vi "toml_api_dump.vi"(7 "resolved path":path, 8 "error in (no error)":errorcluster, 10 "operation (open or create)":T1(ring)=enum."replace or create", 11 "vi in":refnum<vi>) -> (0 "error out":errorcluster, 2 "key exists":bool, 3 "vi out":refnum<vi>)   [LabVIEW 2017]
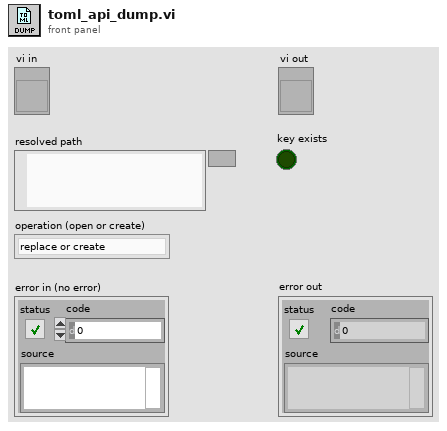
[diagram p1: front panel]
types:
  T1 = enum16{"open", "replace", "create", "open or create", "replace or create", "replace or create with confirmation"}
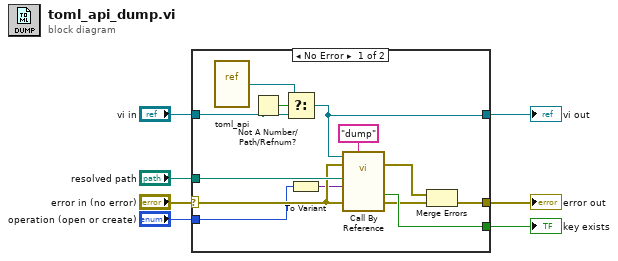
[diagram p0: block diagram]
diagram:
  n1 = case shown="No Error" "error in (no error)" {
    selector: "error in (no error)" -> [w12 w22]
    tunnel: [w20 _] -> w7
    tunnel: "resolved path" -> [w18 _]
    tunnel: [w14 w22] -> w5
    tunnel: "vi in" -> [w11 w21]
    tunnel: [w10 w21] -> w2
    tunnel: "operation (open or create)" -> [w9 _]
    frame No Error {
      n2 = vi-ref "toml_api.vi"() -> (w17:refnum<vi>)
      n3 = Not A Number/Path/Refnum?(number/path/refnum=w11) -> (NaN/Path/Refnum?=w16:bool)
      n4 = Select(t=w17, s=w16, f=w11) -> (s? t:f=w10:refnum<vi>)
      n5 = To Variant(anything=w9) -> (Variant=w8:variant)
      n6 = call-by-ref "?"(reference=w10, error in=w12, "cmd"="dump", 8:"error in (no error)"=w12, "data in"=w8, "path in"=w18) -> (error out=w13:errorcluster, 0:"error out"=w19:errorcluster, "return"=w20:bool)  [unwired: 4 in, 3 out]
      n7 = Merge Errors(w13, w19) -> (w14:errorcluster)
    }
    frame Error {
    }
  }
  "key exists" <- w7
  "error out" <- w5
  "vi out" <- w2
